vi "Read Node Items.vi"(8 "error in (no error)":errorcluster, 11 "Base Tree in":refnum<class "Base Tree.lvclass">) -> (0 "error out":errorcluster, 2 "Node Items":refnum<class "UA Node.lvclass">[](array[class]), 3 "Base Tree out":refnum<class "Base Tree.lvclass">)   [LabVIEW 2017, in "opcua.lvlib" / "Browser Core.lvlib" / "Base Tree.lvclass"]
uses:
  Base Tree.lvclass
  Node Classes/UA Node/UA Node.lvclass
  Base Tree.lvclass/Base Tree.ctl
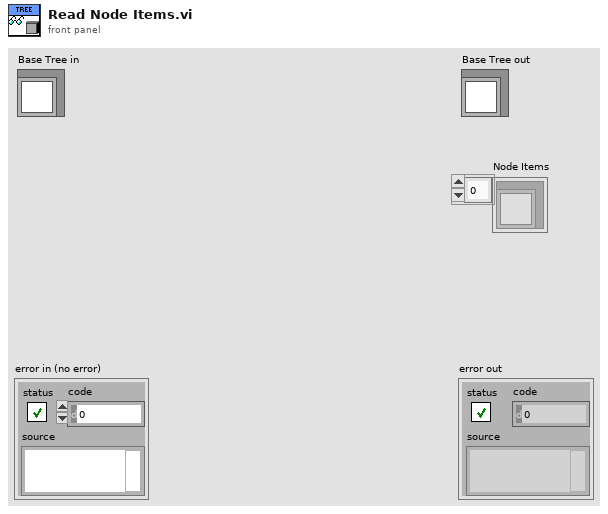
[diagram p1: front panel]
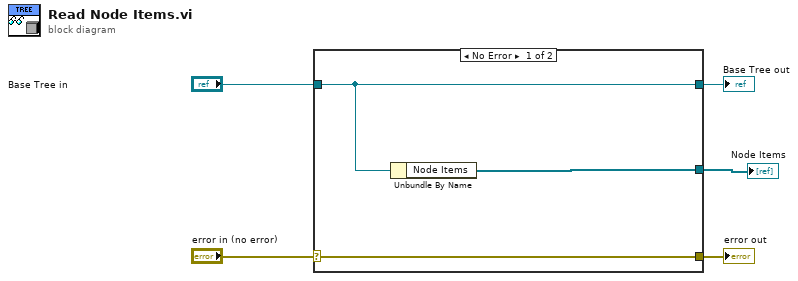
[diagram p0: block diagram]
diagram:
  n1 = case shown="No Error" "error in (no error)" {
    selector: "error in (no error)" -> [w8 w9]
    tunnel: [w8 w9] -> w4
    tunnel: [w7 w10] -> w2
    tunnel: "Base Tree in" -> [w7 w10]
    tunnel: [w6 _] -> w1
    frame No Error {
      n2 = Unbundle By Name(w7) -> ("Node Items"=w6:refnum<class "UA Node.lvclass">[])
    }
    frame Error {
    }
  }
  "error out" <- w4
  "Base Tree out" <- w2
  "Node Items" <- w1
